vi "FRC-Traj-Lib-timer-2-Sample.vi"() -> ()   [LabVIEW 2019]
uses:
  <vilib>/Rock Robotics/WPI/ThirdParty/JAS_Junk/TrajLib/Trajectory_Library.lvlib
panel:
  out "State":i32
  in  "Tab Control":enum32{"Control Panel", "Logic"}(tab)
  in  "Start Timer":bool
  out "Trend":cluster{"CurrentTImer":dbl, "CurrentTImer":dbl}(graph)
  out "Expired":bool
  out "Timer 2":dbl
  out "Timer 1":dbl
  in  "Stop Timer":bool
  # "Timer Sample 2"
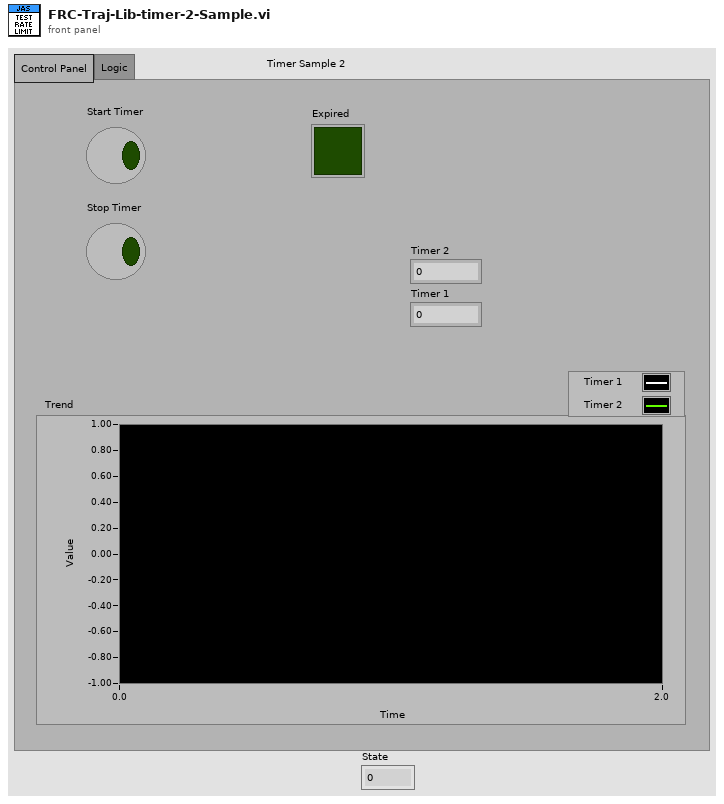
[diagram p1: front panel]
types:
  T1 = typedef "Trajectory_Library.lvlib/TIMER.ctl" = cluster{"StartTime":dbl, "Accumulated TIme":dbl, "Running":bool, "semaphore":T2}
  T2 = typedef "Semaphore RefNum" = refnum<k1>
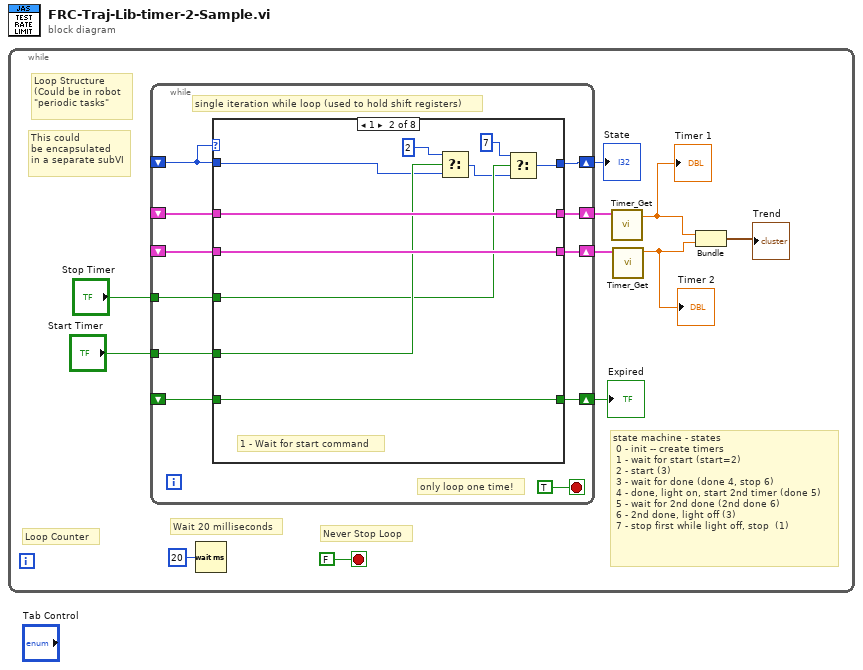
[diagram p0: block diagram]
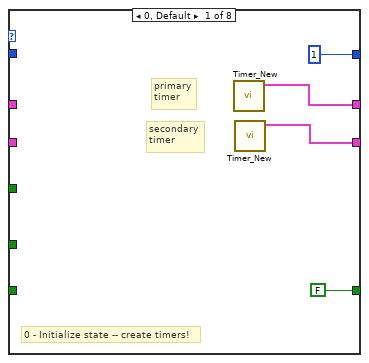
[diagram p2: hidden frame]
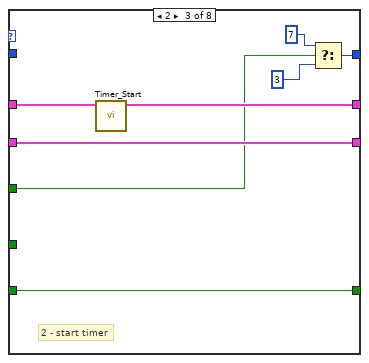
[diagram p3: hidden frame]
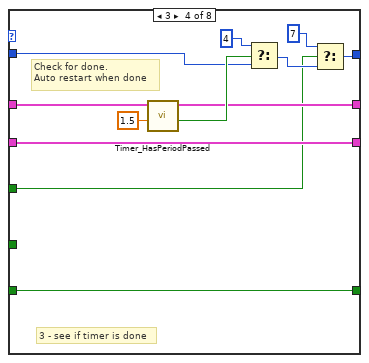
[diagram p4: hidden frame]
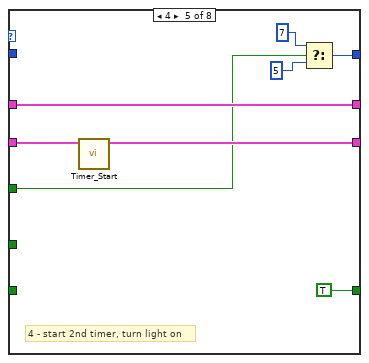
[diagram p5: hidden frame]
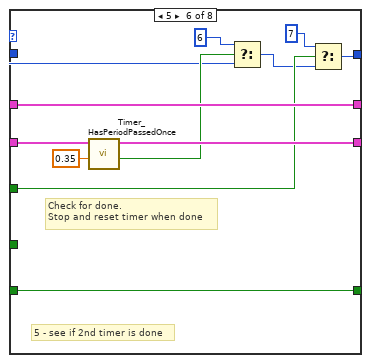
[diagram p6: hidden frame]
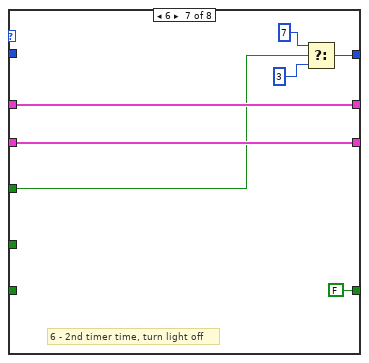
[diagram p7: hidden frame]
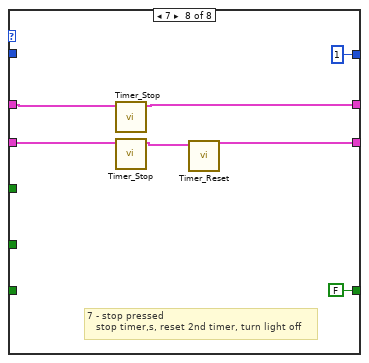
[diagram p8: hidden frame]
diagram:
  n1 = while {
    stop <- FALSE stop-if-true
    # "This could\nbe encapsulated\nin a separate subVI"
    # "Loop Structure\n(Could be in robot\n\"periodic tasks\""
    # "state machine - states\n 0 - init -- create timers\n 1 - wait for start (start=2)\n 2 - start (3)\n 3 - wait for done (done 4, stop 6)\n 4 - done, light on, start 2nd timer (done 5)\n 5 - wait for 2nd done (2nd done 6)\n 6 - 2nd done, light off (3)\n 7 - stop first while light off, stop  (1)"
    # "Loop Counter"
    # "Never Stop Loop"
    # "Wait 20 milliseconds"
    n2 = while {
      shift-right: [w19] -> w9
      shift-left: _ -> [w17]
      shift-right: [w21] -> w6
      shift-left: _ -> [w16]
      shift-right: [w20] -> w5
      shift-left: _ -> [w15]
      tunnel: "Start Timer" -> [w18]
      shift-right: [w14] -> w7
      shift-left: _ -> [w13]
      tunnel: "Stop Timer" -> [w12]
      stop <- TRUE stop-if-true
      # "only loop one time!"
      # "single iteration while loop (used to hold shift registers)"
      n3 = case shown="1" w17 {
        tunnel: [w26 w36 w43 w52 w64 w76 w82 w85] -> w21
        tunnel: [w25 w35 w42 w50 w62 w72 w81 w86] -> w20
        tunnel: [1 w27 w37 w45 w59 w67 w78 1 ("t")] -> w19
        tunnel: w18 -> [_ w34 _ _ _ _ _ _]
        tunnel: w17 -> [_ w33 _ w51 _ w69 _ _]
        tunnel: w16 -> [_ w36 w44 w53 w64 w76 w82 w89]
        tunnel: w15 -> [_ w35 w42 w50 w63 w73 w81 w88]
        tunnel: [FALSE w31 w41 w49 TRUE w75 FALSE FALSE] -> w14
        tunnel: w13 -> [_ w31 w41 w49 _ w75 _ _]
        tunnel: w12 -> [_ w29 w38 w46 w57 w66 w77 _]
        frame 0, Default {
          # "0 - Initialize state -- create timers!"
          # "secondary\ntimer"
          # "primary\ntimer"
          n4 = call <vilib>:"Timer_New.vi"() -> ("TIMER"=w26:T1)  [unwired: 11 in]
          n5 = call <vilib>:"Timer_New.vi"() -> ("TIMER"=w25:T1)  [unwired: 11 in]
        }
        frame 1 {
          # "1 - Wait for start command"
          n6 = Select(t=2, s=w34, f=w33) -> (s? t:f=w28:i32)
          n7 = Select(t=7, s=w29, f=w28) -> (s? t:f=w27:i32)
        }
        frame 2 {
          # "2 - start timer"
          n8 = call <vilib>:"Timer_Start.vi"("in Timer"=w44) -> ("out Timer"=w43:T1)  [unwired: 10 in]
          n9 = Select(t=7, s=w38, f=3) -> (s? t:f=w37:i32)
        }
        frame 3 {
          # "Check for done.\nAuto restart when done"
          # "3 - see if timer is done"
          n10 = call <vilib>:"Timer_HasPeriodPassed.vi"("Period"=1.5, "in Timer"=w53) -> ("Expired"=w54:bool, "out Timer"=w52:T1)  [unwired: 7 in, 1 out]
          n11 = Select(t=4, s=w54, f=w51) -> (s? t:f=w47:i32)
          n12 = Select(t=7, s=w46, f=w47) -> (s? t:f=w45:i32)
        }
        frame 4 {
          # "4 - start 2nd timer, turn light on"
          n13 = call <vilib>:"Timer_Start.vi"("in Timer"=w63) -> ("out Timer"=w62:T1)  [unwired: 10 in]
          n14 = Select(t=7, s=w57, f=5 ("t")) -> (s? t:f=w59:i32)
        }
        frame 5 {
          # "Check for done.\nStop and reset timer when done"
          # "5 - see if 2nd timer is done"
          n15 = call <vilib>:"Timer_HasPeriodPassedOnce.vi"("Period"=0.35, "in Timer"=w73) -> ("Expired"=w70:bool, "out Timer"=w72:T1)  [unwired: 7 in, 1 out]
          n16 = Select(t=6, s=w70, f=w69) -> (s? t:f=w65:i32)
          n17 = Select(t=7, s=w66, f=w65) -> (s? t:f=w67:i32)
        }
        frame 6 {
          # "6 - 2nd timer time, turn light off"
          n18 = Select(t=7, s=w77, f=3 ("t")) -> (s? t:f=w78:i32)
        }
        frame 7 {
          # "7 - stop pressed\n   stop timer,s, reset 2nd timer, turn light off"
          n19 = call <vilib>:"Timer_Stop.vi"("in Timer"=w89) -> ("out Timer"=w85:T1)  [unwired: 10 in]
          n20 = call <vilib>:"Timer_Stop.vi"("in Timer"=w88) -> ("out Timer"=w87:T1)  [unwired: 10 in]
          n21 = call <vilib>:"Timer_Reset.vi"("in TIMER"=w87) -> ("out TIMER"=w86:T1)  [unwired: 10 in]
        }
      }
    }
    "Expired" <- w7
    "State" <- w9
    n22 = Wait (ms)(milliseconds to wait=u32 20) -> ()  [unwired: 1 out]
    n23 = call <vilib>:"Timer_Get.vi"("TIMER"=w6) -> ("CurrentTImer"=w4:dbl)  [unwired: 10 in]
    "Timer 1" <- w4
    n24 = call <vilib>:"Timer_Get.vi"("TIMER"=w5) -> ("CurrentTImer"=w3:dbl)  [unwired: 10 in]
    "Timer 2" <- w3
    n25 = Bundle("CurrentTImer"=w4, "CurrentTImer"=w3) -> (→"Trend":cluster{"CurrentTImer":dbl, "CurrentTImer":dbl})  [unwired: 1 in]
  }
